vi "TRAJECTORY_FGV.vi"(9 "inTRAJECTORY":T1 {"States"."POSE"."ROTATION"."SIN" format="%13.4f"; "States"."POSE"."ROTATION"."COS" format="%13.4f"; "States"."POSE"."ROTATION"."VALUE" format="%13.4f"; "States"."POSE"."TRANSLATION"."Y" format="%14.3f"; "States"."POSE"."TRANSLATION"."X" format="%14.3f"; "TotalTImeSecs" format="%20.3f"}, 11 "WRITE":bool) -> (1 "outTRAJECTORY":T1 {"States"."POSE"."ROTATION"."SIN" format="%13.4f"; "States"."POSE"."ROTATION"."COS" format="%13.4f"; "States"."POSE"."ROTATION"."VALUE" format="%13.4f"; "States"."POSE"."TRANSLATION"."Y" format="%14.3f"; "States"."POSE"."TRANSLATION"."X" format="%14.3f"; "TotalTImeSecs" format="%20.3f"})   [LabVIEW 2019]
uses:
  <vilib>/Rock Robotics/WPI/ThirdParty/JAS_Junk/TrajLib/TypeDef/TRAJECTORY.ctl
  <vilib>/Rock Robotics/WPI/ThirdParty/JAS_Junk/TrajLib/TypeDef/TRAJ_STATE.ctl
  <vilib>/Rock Robotics/WPI/ThirdParty/JAS_Junk/TrajLib/TypeDef/POSE2D.ctl
  <vilib>/Rock Robotics/WPI/ThirdParty/JAS_Junk/TrajLib/TypeDef/TRANSLATION2D.ctl
  <vilib>/Rock Robotics/WPI/ThirdParty/JAS_Junk/TrajLib/TypeDef/ROTATION2D.ctl
  <vilib>/Rock Robotics/WPI/ThirdParty/JAS_Junk/TrajLib/Trajectory_Library.lvlib
panel:
  # "This is purposefully \n\nNOT re-entrant."
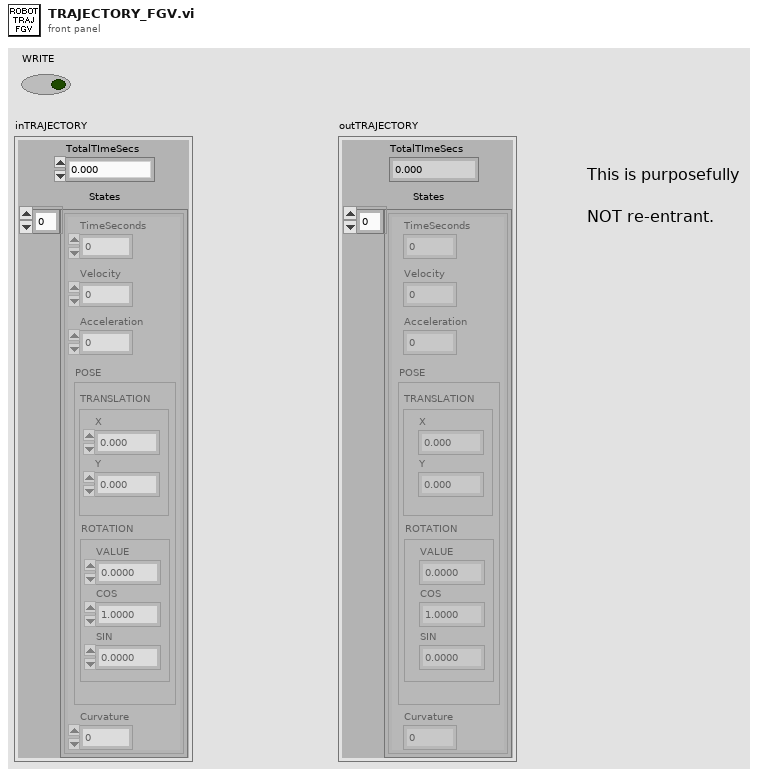
[diagram p1: front panel]
types:
  T1 = typedef "Trajectory_Library.lvlib/TRAJECTORY.ctl" = cluster{"TotalTImeSecs":dbl, "States":T2[]}
  T2 = typedef "Trajectory_Library.lvlib/TRAJ_STATE.ctl" = cluster{"TimeSeconds":dbl, "Velocity":dbl, "Acceleration":dbl, "POSE":T3, "Curvature":dbl}
  T3 = typedef "Trajectory_Library.lvlib/POSE2D.ctl" = cluster{"TRANSLATION":T4, "ROTATION":T5}
  T4 = typedef "Trajectory_Library.lvlib/TRANSLATION2D.ctl" = cluster{"X":dbl, "Y":dbl}
  T5 = typedef "Trajectory_Library.lvlib/ROTATION2D.ctl" = cluster{"VALUE":dbl, "COS":dbl, "SIN":dbl}
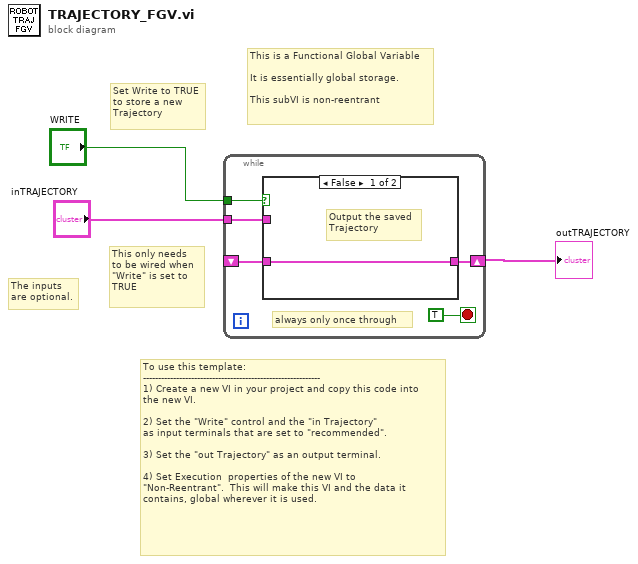
[diagram p0: block diagram]
diagram:
  # "This only needs\nto be wired when\n\"Write\" is set to\nTRUE"
  # "To use this template:\n-----------------------------------------------------------\n1) Create a new VI in your project and copy this code into\nthe new VI.\n\n2) Set the \"Write\" control and the \"in Trajectory\"\nas input terminals that are set to \"recommended\".\n\n3) Set the \"out Trajectory\" as an output terminal.\n\n4) Set Execution  properties of the new VI to \n\"Non-Reentrant\".  This will make this VI and the data it \ncontains, global wherever it is used."
  # "Set Write to TRUE\nto store a new\nTrajectory"
  # "The inputs \nare optional."
  # "This is a Functional Global Variable\n\nIt is essentially global storage.\n\nThis subVI is non-reentrant"
  n1 = while {
    tunnel: "WRITE" -> [w7]
    tunnel: "inTRAJECTORY" -> [w5]
    shift-right: [w6] -> w3
    shift-left: _ -> [w4]
    stop <- TRUE stop-if-true
    # "always only once through"
    n2 = case shown="False" w7 {
      tunnel: [w9 w10] -> w6
      tunnel: w5 -> [_ w10]
      tunnel: w4 -> [w9 _]
      frame False {
        # "Output the saved\nTrajectory"
      }
      frame True {
        # "Save the trajectory\nin the shift \nregister."
      }
    }
  }
  "outTRAJECTORY" <- w3
